vi "go to floor.vi"(2 "current floor in":dbl, 4 "floor cluster in":T1) -> (0 "new floor out":dbl, 1 "state out":T2)   [LabVIEW 2020]
uses:
  state.ctl
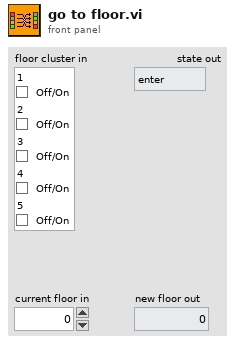
[diagram p1: front panel]
types:
  T1 = cluster{"1":bool, "2":bool, "3":bool, "4":bool, "5":bool}
  T2 = typedef "state.ctl" = enum16{"enter", "checking", "go up", "go down", "process", "get out", "temp"}
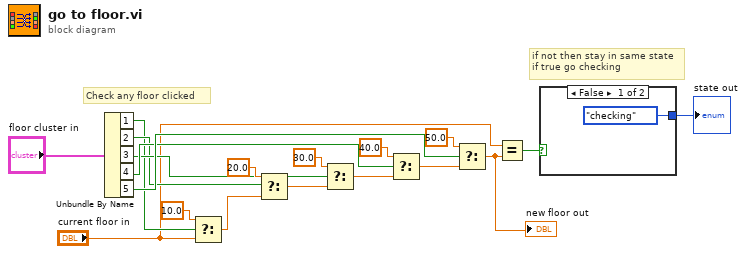
[diagram p0: block diagram]
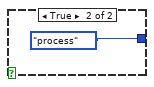
[diagram p2: hidden frame]
diagram:
  # "if not then stay in same state\nif true go checking"
  # "Check any floor clicked"
  n1 = Unbundle By Name("floor cluster in") -> ("1"=w5:bool, "2"=w6:bool, "3"=w7:bool, "4"=w8:bool, "5"=w9:bool)
  n2 = Select(t=10.0, s=w5, f="current floor in") -> (s? t:f=w13:dbl)
  n3 = Select(t=20.0, s=w6, f=w13) -> (s? t:f=w12:dbl)
  n4 = Select(t=30.0, s=w7, f=w12) -> (s? t:f=w11:dbl)
  n5 = Select(t=40.0, s=w8, f=w11) -> (s? t:f=w10:dbl)
  n6 = Select(t=50.0, s=w9, f=w10) -> (s? t:f=w2:dbl)
  "new floor out" <- w2
  n7 = Equal?(x="current floor in", y=w2) -> (x = y?=w3:bool)
  n8 = case shown="False" w3 {
    tunnel: [state."checking" state."process"] -> w4
    frame False {
    }
    frame True {
    }
  }
  "state out" <- w4
